vi "manipulate simulated data.vi"() -> ()   [LabVIEW 2016]
uses:
  <vilib>/Analysis/NI_AALBase.lvlib
  <vilib>/Analysis/NI_AALPro.lvlib
panel:
  out "reversed array":cluster{dbl[], dbl[]}[](graph)
  in  "length 2":i32=197
  in  "index 4":i32
  in  "device B":cluster{dbl[], dbl[]}[](graph)
  in  "device D":cluster{dbl[], dbl[]}[](graph)
  out "FWHM":dbl=141.55902502562543
  out "input G 9":cluster{dbl[], dbl[]}(graph)
  in  "length":i32=65
  in  "index 3":i32=19
  out "result":dbl=3.000700892436365
  in  "w":dbl=0.03 format="%#_13g"
  in  "V":dbl=0.318 format="%#_13g"
  in  "A":dbl=1.0 format="%#_13g"
  out "input G 8":cluster{dbl[], dbl[]}(graph)
  in  "Numeric":dbl=3.0
  in  "index 2":i32=53
  out "input G 7":cluster{dbl[], dbl[]}(graph)
  out "input G 6":cluster{dbl[], dbl[]}[](graph)
  in  "index":i32=21
  in  "input G 5":cluster{dbl[], dbl[]}[](graph)
  out "size(s)":i32=100
  out "input G 4":cluster{dbl[], dbl[]}[](graph)
  in  "Min G":dbl
  in  "Max G":dbl=8.5
  in  "input G 3":cluster{dbl[], dbl[]}[](graph)
  out "input G 2":cluster{dbl[], dbl[]}[](graph)
  in  "amplitude":dbl=0.005 format="%0.2f"
  in  "input G":cluster{dbl[], dbl[]}[](graph)
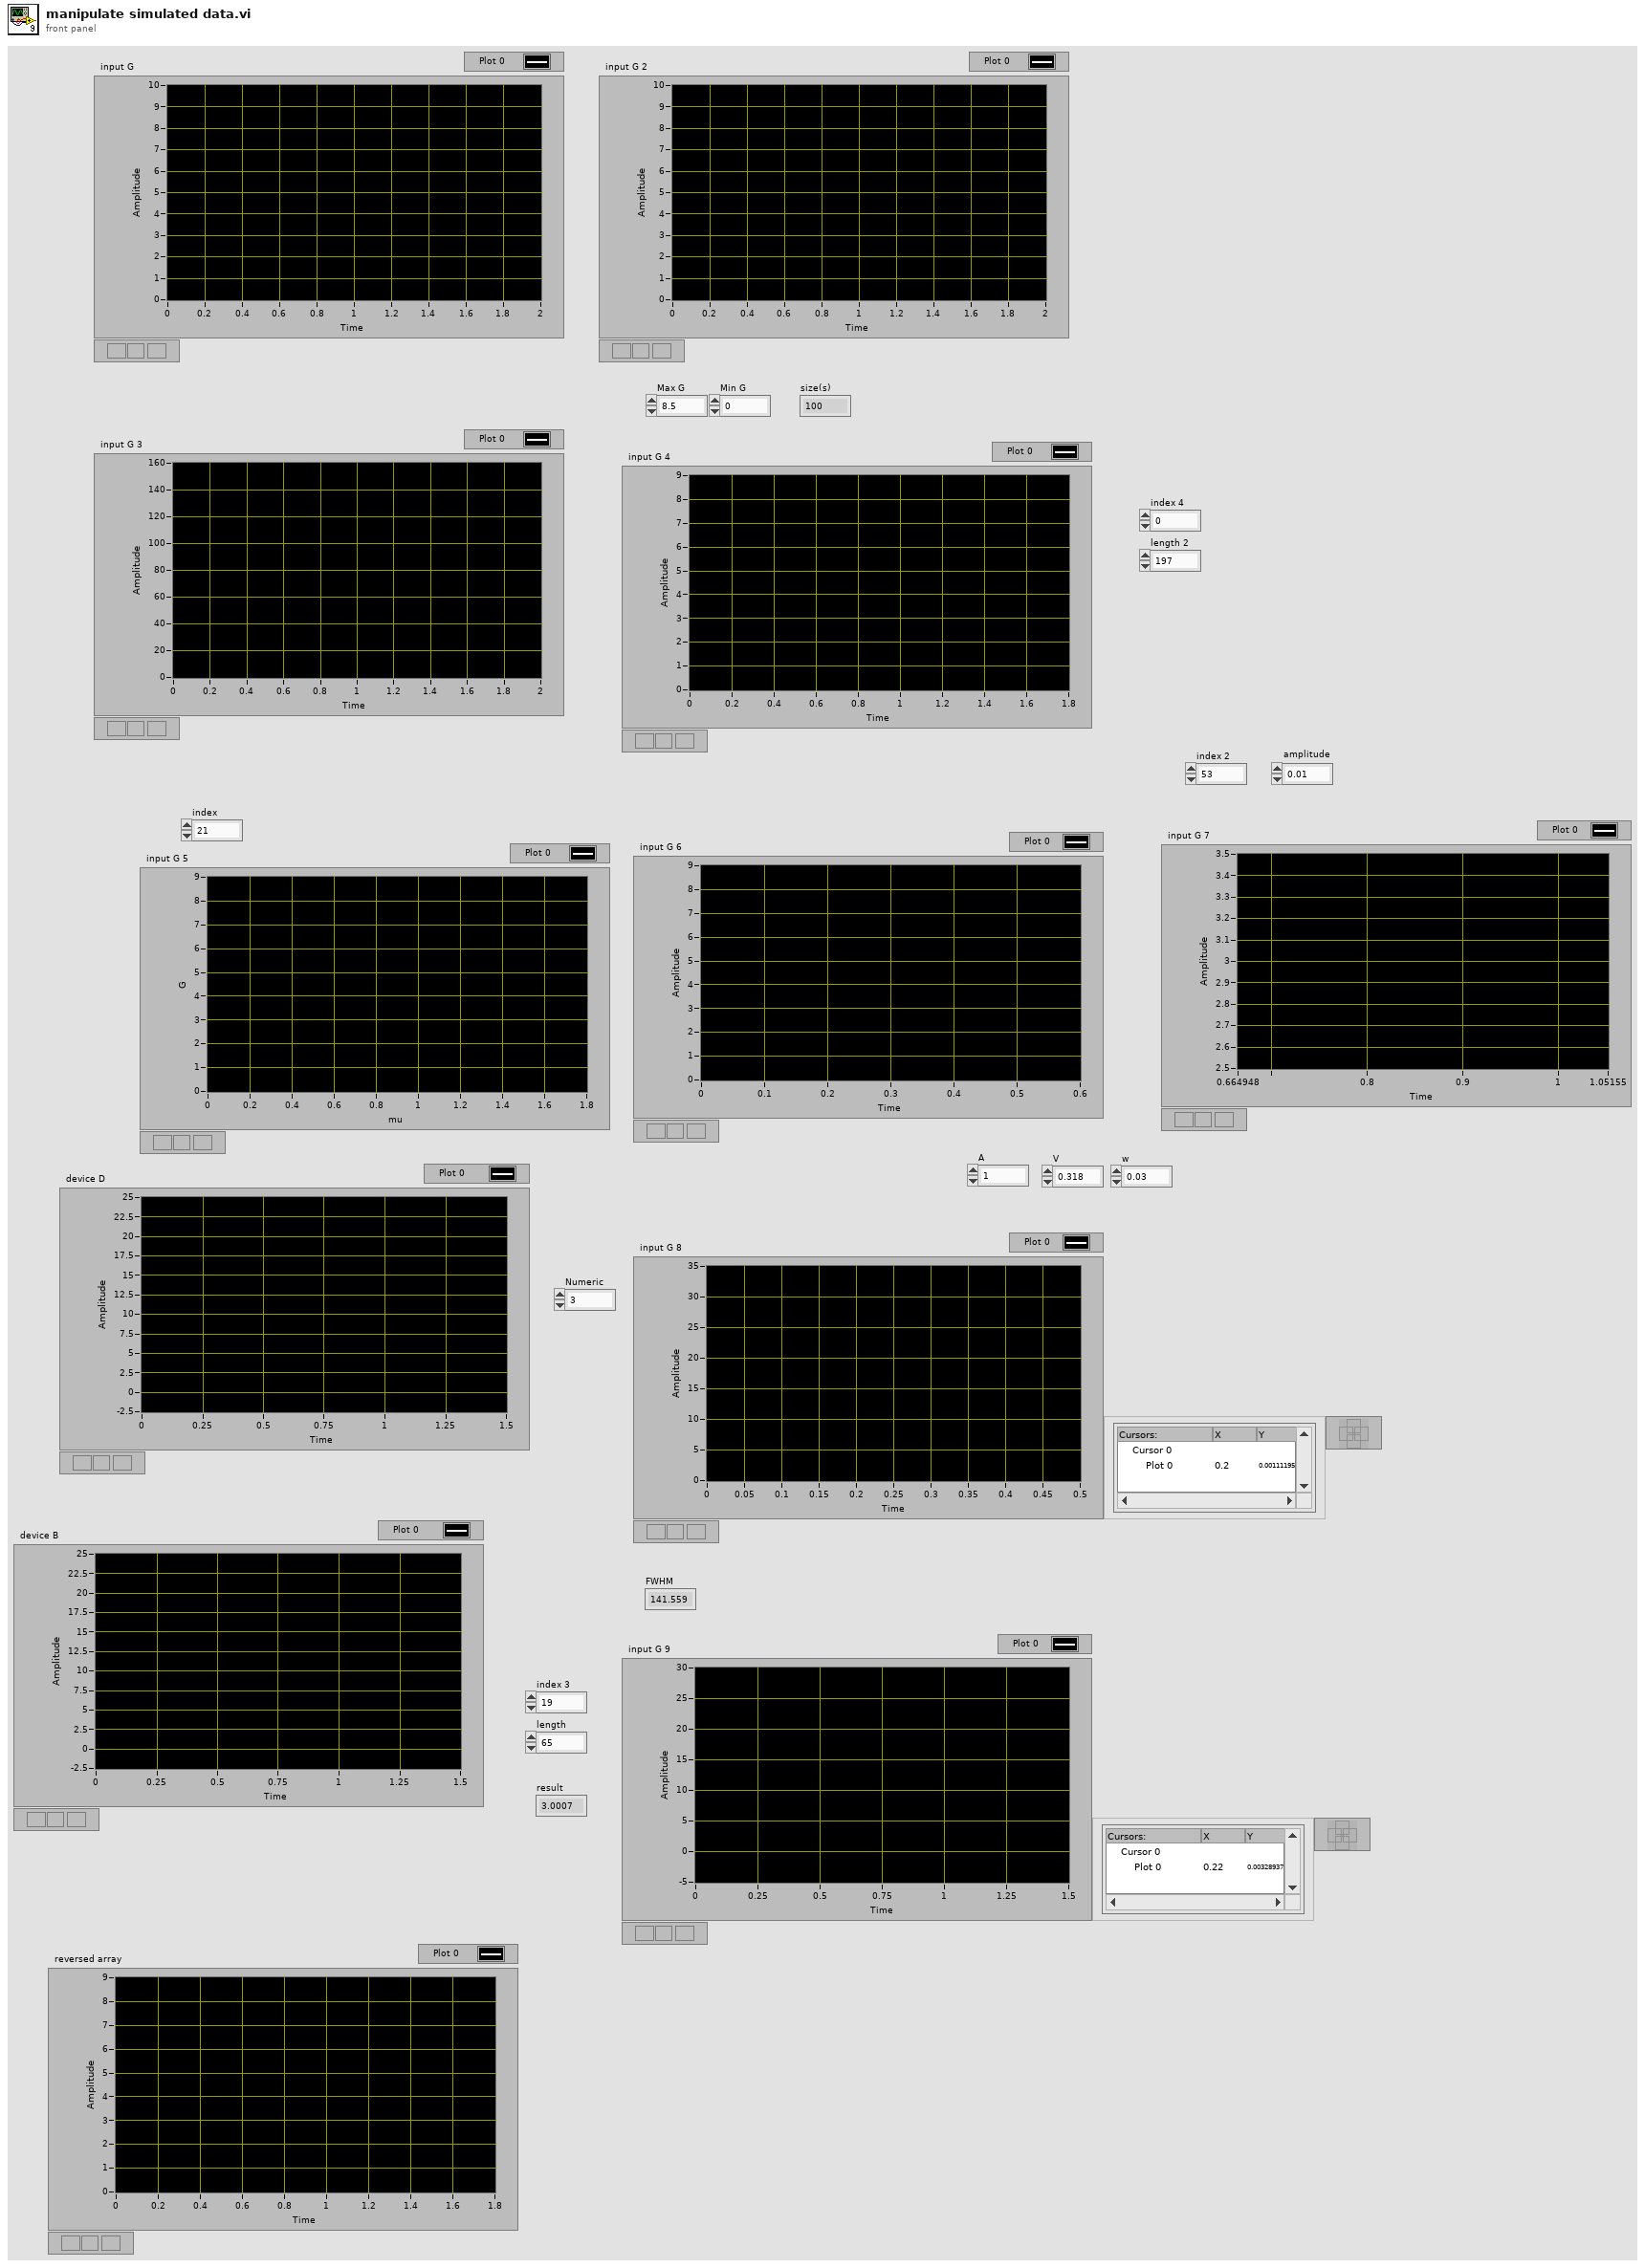
[diagram p1: front panel]
types:
  T1 = cluster{"Decimated Array":dbl[], "Decimated Array":dbl[]}
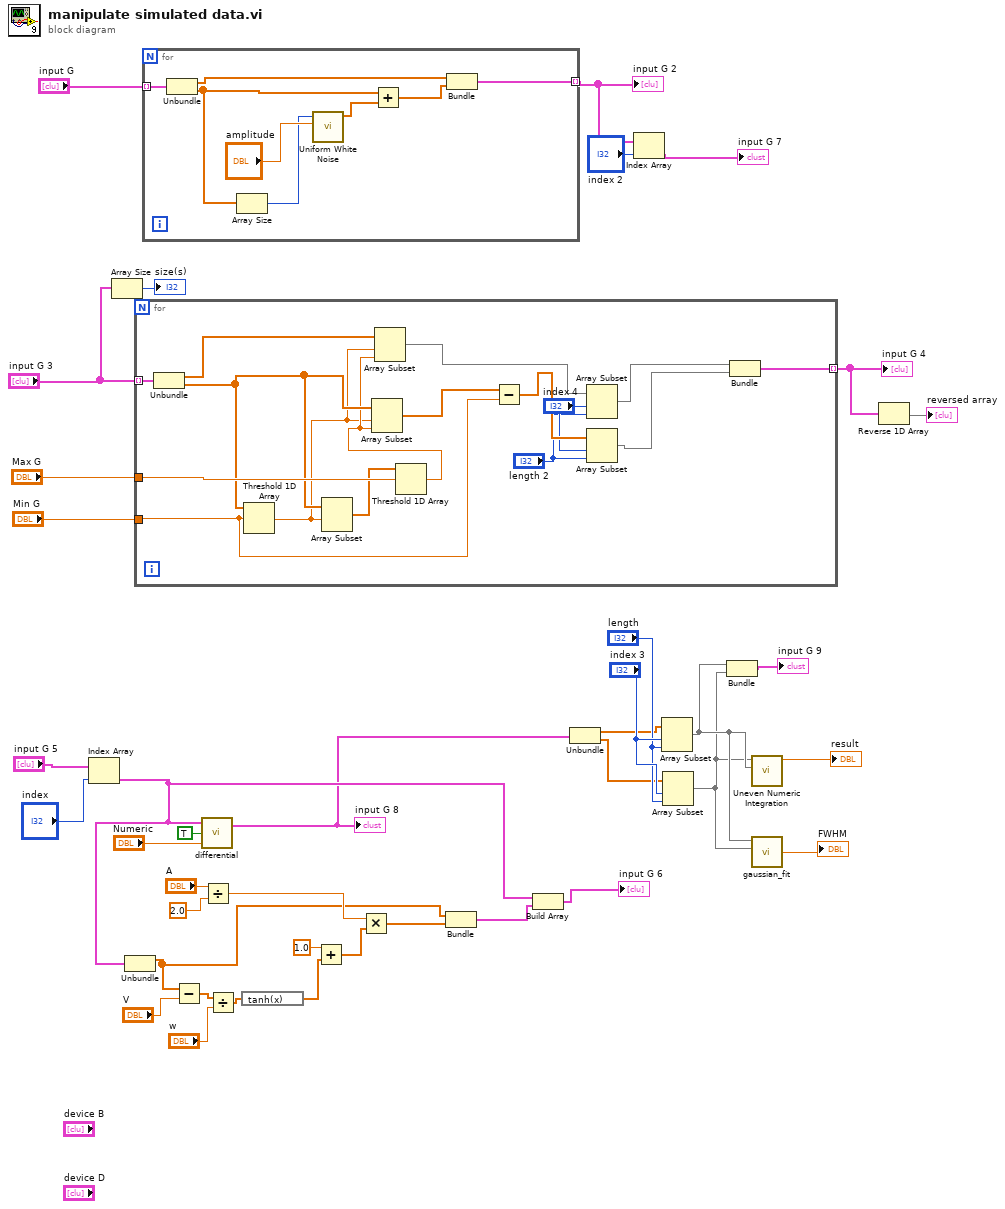
[diagram p0: block diagram]
diagram:
  n1 = Index Array(array="input G 5", index="index") -> (element=w17:cluster{dbl[], dbl[]})
  n2 = Array Size(array="input G 3") -> (size(s)=→"size(s)":i32)
  n3 = Unbundle(w17) -> (w13:dbl[])  [unwired: 1 out]
  n4 = for {
    tunnel: "input G 3" -> [w55] mode=indexing
    tunnel: "Max G" -> [w54]
    tunnel: "Min G" -> [w46]
    tunnel: [w52] -> w2 mode=indexing
    n5 = Unbundle(w55) -> (w53:dbl[], w51:dbl[])
    n6 = Threshold 1D Array(2:w46, 3:w51) -> (0:w47:dbl)  [unwired: 1 in]
    n7 = Array Subset(array=w51, index=w47) -> (w50:dbl[])  [unwired: 1 in]
    n8 = Threshold 1D Array(2:w54, 3:w50) -> (0:w49:dbl)  [unwired: 1 in]
    n9 = Array Subset(array=w51, index=w47, length=w49) -> (w48:dbl[])
    n10 = Array Subset(array=w53, index=w47, length=w49) -> (w45:dbl[])
    n11 = Subtract(x=w48, y=w46) -> (x-y=w44:dbl[])
    n12 = Array Subset(array=w45, index="index 4", length="length 2") -> (w40:dbl[])
    n13 = Array Subset(array=w44, index="index 4", length="length 2") -> (w41:dbl[])
    n14 = Bundle(w40, w41) -> (w52:cluster{dbl[], dbl[]})  [unwired: 1 in]
  }
  "input G 4" <- w2
  n15 = for {
    tunnel: "input G" -> [w63] mode=indexing
    tunnel: [w56] -> w32 mode=indexing
    n16 = Unbundle(w63) -> (w58:dbl[], w60:dbl[])
    n17 = Array Size(array=w60) -> (size(s)=w59:i32)
    n18 = call <vilib>:"Uniform White Noise.vi"("amplitude"="amplitude", "samples"=w59) -> ("uniform white noise"=w62:dbl[])  [unwired: 8 in, 1 out]
    n19 = Add(x=w60, y=w62) -> (x+y=w57:dbl[])
    n20 = Bundle(w58, w57) -> (w56:cluster{dbl[], dbl[]})  [unwired: 1 in]
  }
  "input G 2" <- w32
  n21 = Subtract(x=w13, y="V") -> (x-y=w22:dbl[])
  n22 = call <userlib>:"differential.vi"("Numeric"="Numeric", "dy/dx vs x"=TRUE, "A vs B 2"=w17) -> ("A vs B 3"=w12:T1)  [unwired: 1 in]
  "input G 8" <- w12
  n23 = Divide(x="A", y=2.0) -> (x/y=w25:dbl)
  n24 = Divide(x=w22, y="w") -> (x/y=w15:dbl[])
  n25 = expression code="tanh(x)"(w15) -> (w14:dbl[])
  n26 = Add(x=1.0, y=w14) -> (x+y=w20:dbl[])
  n27 = Multiply(x=w25, y=w20) -> (x*y=w19:dbl[])
  n28 = Bundle(w13, w19) -> (w18:cluster{dbl[], dbl[]})  [unwired: 1 in]
  n29 = Build Array(w17, w18) -> (→"input G 6":cluster{dbl[], dbl[]}[])
  n30 = Unbundle(w12) -> ("Decimated Array"=w6:dbl[], "Decimated Array"=w7:dbl[])
  n31 = Index Array(array=w32, index="index 2") -> (element=→"input G 7":cluster{dbl[], dbl[]})
  n32 = Array Subset(array=w6, index="index 3", length="length") -> (w5:dbl[])
  n33 = Array Subset(array=w7, index="index 3", length="length") -> (w4:dbl[])
  n34 = Bundle(w5, w4) -> (→"input G 9":cluster{dbl[], dbl[]})  [unwired: 1 in]
  n35 = call <vilib>:"Uneven Numeric Integration.vi"("T"=w5, "X"=w4) -> ("result"=→"result":dbl)  [unwired: 8 in, 1 out]
  n36 = call "gaussian_fit.vi"("Y Values"=w4, "X Values"=w5) -> ("FWHM"=→"FWHM":dbl)  [unwired: 2 in, 5 out]
  n37 = Reverse 1D Array(array=w2) -> (reversed array=→"reversed array":cluster{dbl[], dbl[]}[])
